vi "Measurement Logic.vi"(8 "error in":errorcluster, 9 "measurement configuration":T4={"config"="SI1", "BITFILE"=""}, 10 "measure call context in":refnum<class "Measure Call Context.lvclass">, 11 "user event out":refnum<user-event>) -> (0 "Error Out":errorcluster, 2 "measure call context out":refnum<class "Measure Call Context.lvclass">, 3 "measurement results":T1 {"BYTES ACQUIRED" format="%#.6p"})   [LabVIEW 2025, in "Automotive Vision.lvclass"]
doc: "Contains the core logic for executing the measurement."
uses:
  Automotive Vision.lvclass
  <vilib>/Plug-In SDKs/Measurements/Measure Call Context/Measure Call Context.lvclass
  <vilib>/rvi/interface/nirviCloseFPGA/nirviCloseFPGA.xnode
  Measurement Results.ctl
  <vilib>/FPGAPlugInAG/Dynamic/niLvFpga_Close_Dynamic.vi
  ttashjia/GSE/Host/Acq/GettingStarted_Acq_148X_Host.lvlib
  ttashjia/GSE/Host/Common/GettingStarted_Common_148X_Host.lvlib
  <instrlib>/FlexRIO/API/Host/v1/NI FlexRIO API v1.lvlib
  <vilib>/vision/Image Controls.llb/IMAQ Image.ctl
  <instrlib>/FlexRIO/CSI-2/v2/Common/Types/LLP Data Type.ctl
  <instrlib>/FlexRIO/CSI-2/v2/Common/NI CSI-2 API Common v2.lvlib
  <instrlib>/FlexRIO/API/Host/v1/NI FlexRIO/API/Wait for PoC Safe to Disconnect Channels Array.vi
  Measurement Configuration.ctl
panel:
  in  "Serial Channel (2nd Display)":fxp<+,3,3>
  in  "Serial Channel (1st Display)":fxp<+,3,3>
  in  "Acquired Serial Input Channel Data":T2(tab)
  out "Source Rate (fps)(1st Display)":dbl
  out "Update Rate (fps)(1st Display)":dbl
  out "1st channel display":T3(plugin-control)
  out "Bytes Acquired (1st Channel)":i64 format="%#.6p"
  out "Packets Logged (1st Channel)":i64
  out "Source Rate (fps)(2nd Display)":dbl
  out "Update Rate (fps)(2nd Display)":dbl
  out "2nd channel display":T3(plugin-control)
  out "Packets Logged (2nd Channel)":i64
  out "Bytes Acquired (2nd Channel)":i64 format="%#.6p"
  out "Acquisition In Progress":bool
  out "Acquisition Duration (s)":dbl format="%.1f"
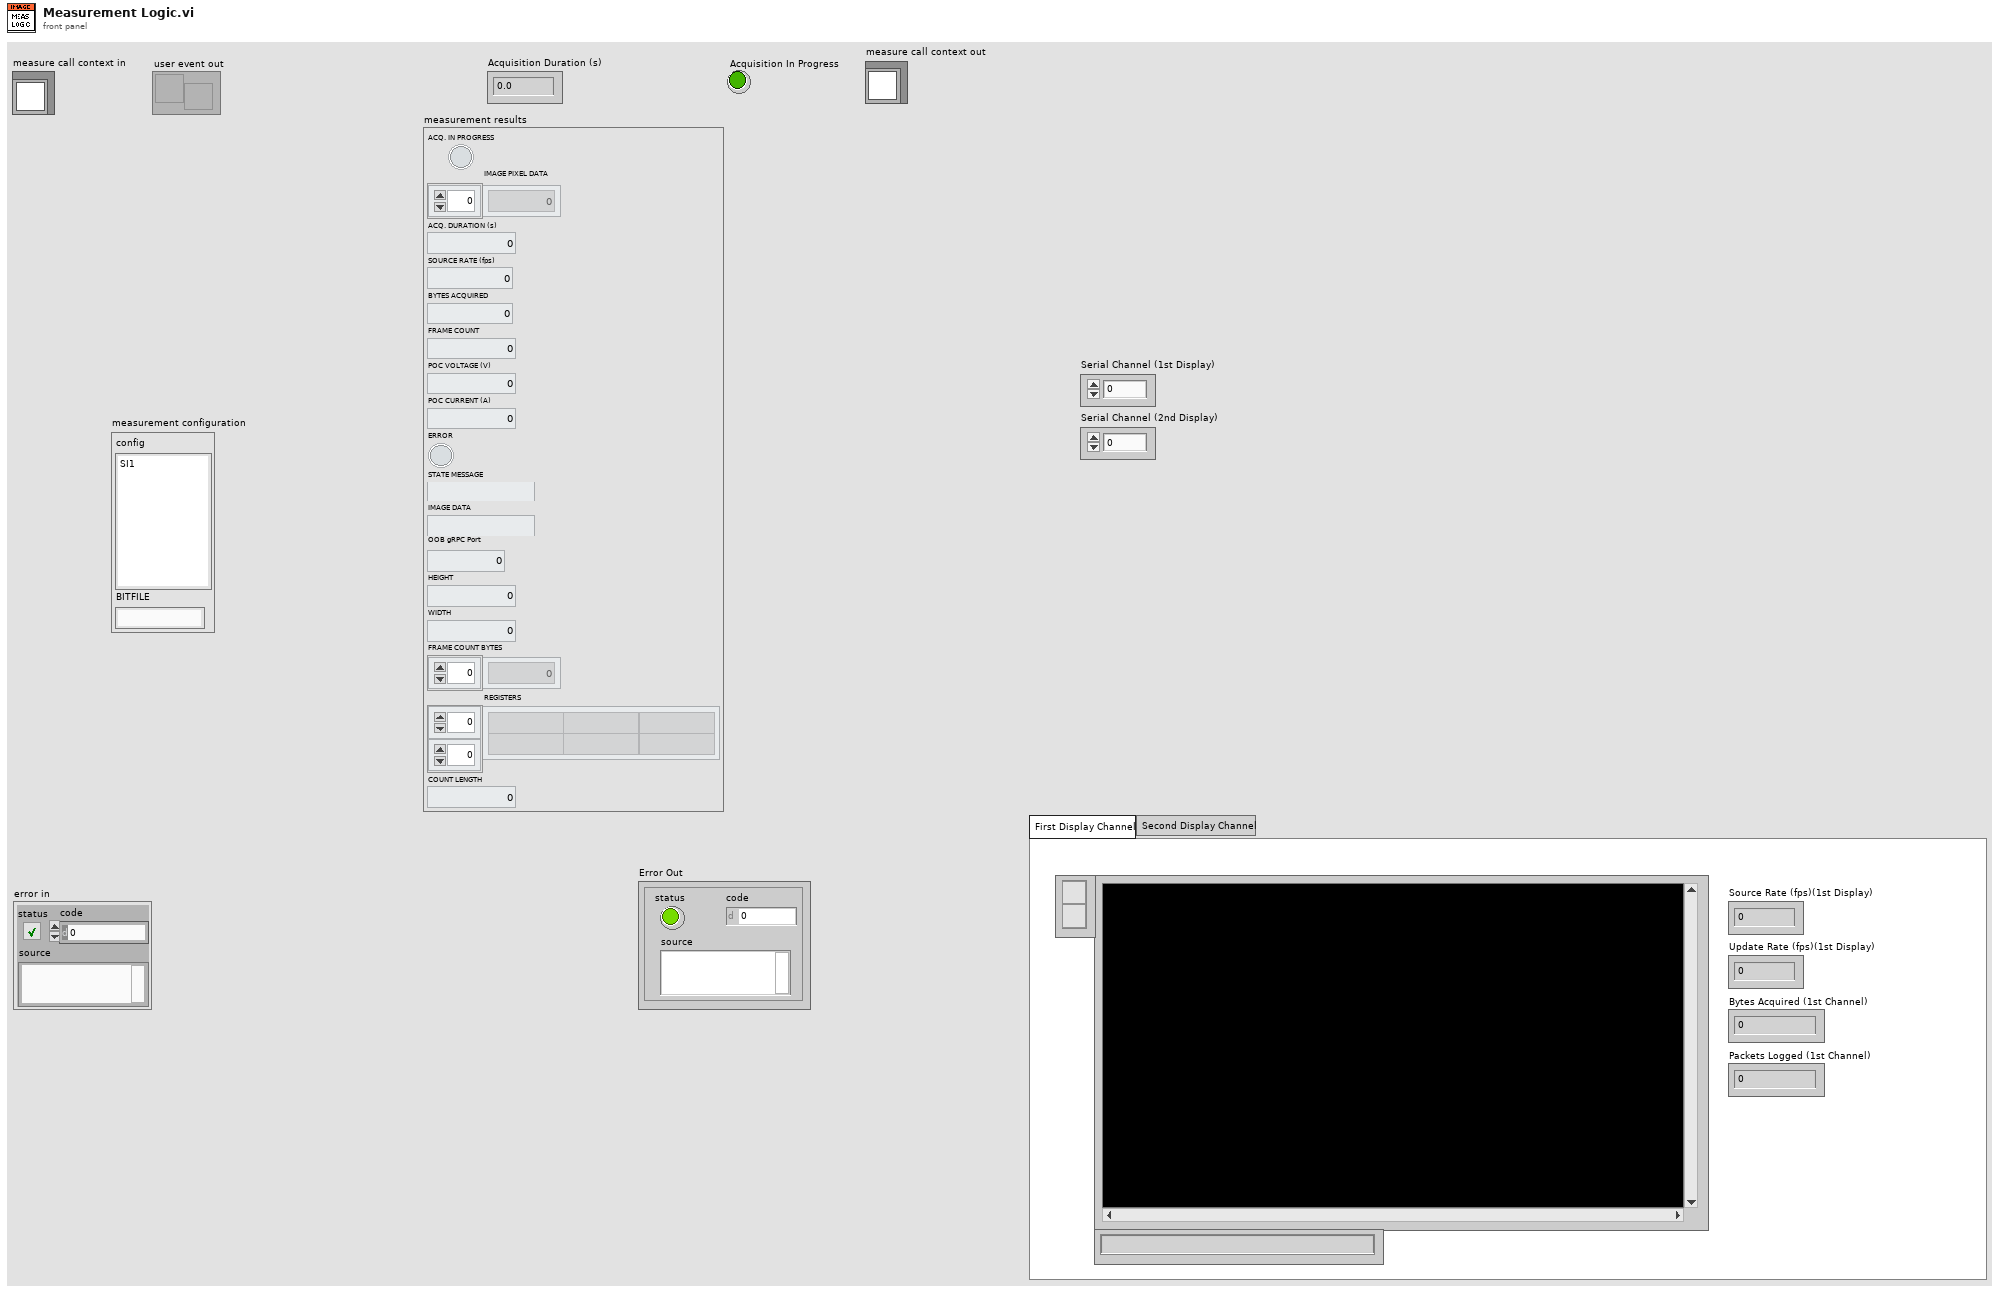
[diagram p1: front panel]
types:
  T1 = typedef "Automotive Vision.lvclass/Measurement Results.ctl" = cluster{"ACQ. IN PROGRESS":bool, "IMAGE PIXEL DATA":u32[], "ACQ. DURATION (s)":dbl, "SOURCE RATE (fps)":dbl, "BYTES ACQUIRED":u64, "FRAME COUNT":u64, "POC VOLTAGE (V)":dbl, "POC CURRENT (A)":dbl, "ERROR":bool, "STATE MESSAGE":string, "IMAGE DATA":string, "OOB gRPC Port":i32, "HEIGHT":u64, "WIDTH":u64, "FRAME COUNT BYTES":u32[], "REGISTERS":string[][], "COUNT LENGTH":u64}
  T2 = enum32{"First Display Channel", "Second Display Channel"}
  T3 = typedef "IMAQ Image.ctl" = refnum<image>
  T4 = typedef "Automotive Vision.lvclass/Measurement Configuration.ctl" = cluster{"config":string, "BITFILE":string}
  T5 = typedef "NI CSI-2 API Common v2.lvlib/LLP Data Type.ctl" = enum8{"Frame Start", "Frame End", "Line Start", "Line End", "End of Transmission", "Reserved 0", "Reserved 1", "Reserved 2", "Generic Short Packet 1", "Generic Short Packet 2", "Generic Short Packet 3", "Generic Short Packet 4", "Generic Short Packet 5", "Generic Short Packet 6", "Generic Short Packet 7", "Generic Short Packet 8", "Null", "Blanking Data", "Embedded 8-bit non Image Data", "Generic Long Packet 1", "Generic Long Packet 2", "Generic Long Packet 3", "Generic Long Packet 4", "Reserved 3", "YUV420 8-bit", "YUV420 10-bit", "Legacy YUV420 8-bit", "Reserved 4", "YUV420 8-bit Chroma Shifted", "YUV420 10-bit Chroma Shifted", "YUV422 8-bit", "YUV422 10-bit", "RGB444", "RGB555", "RGB565", "RGB666", "RGB888", "Reserved 5", "Reserved 6", "RAW 24", "RAW 6", "RAW 7", "RAW 8", "RAW 10", "RAW 12", "RAW 14", "RAW 16", "RAW 20", "User Defined 8-bit Data 1", "User Defined 8-bit Data 2", "User Defined 8-bit Data 3", "User Defined 8-bit Data 4", "User Defined 8-bit Data 5", "User Defined 8-bit Data 6", "User Defined 8-bit Data 7", "User Defined 8-bit Data 8", "USL Command", "Reserved 7", "Reserved 8", "Reserved 9", "Reserved 10", "Reserved 11", "Reserved 12", "LRTE EPD Spacer"}
  T6 = typedef "GettingStarted_Common_148X_Host.lvlib/Serial Channel Configuration.ctl" = cluster{"Serial Channel":string, "FPGA Display Parameters":T7, "RAW Display Parameters":cluster{"Interpretation":T8, "Bayer Parameters":cluster{"Pattern":i32, "Algorithm":i32, "Red Gain":dbl, "Green Gain":dbl, "Blue Gain":dbl}}}
  T7 = typedef "NI CSI-2 API FPGA v2.lvlib/Display Parameters.ctl" = cluster{"virtual channel":fxp<+,4,4>, "payload data type":T5, "frame skip count":u16, "line skip count":u8, "pixel skip count":fxp<+,5,5>}
  T8 = typedef "GettingStarted_Common_148X_Host.lvlib/RAW Interpretation for Display.ctl" = enum16{"Grayscale", "Bayer", "RGB", "YUV422", "YUV420", "Legacy YUV420"}
  T9 = typedef "Automotive Vision.lvclass/autovision_config.ctl" = cluster{"RIO Device":string, "Serial Channel":string, "SERDES Script":string, "POC Source":u32, "CSI-2 Data Source":u32, "Lane Count":u32, "Reference Clock":dbl, "Image Data Type":u32, "Interpretation":u32, "Pattern":u32, "Algorithm":u32, "Virtual Channel":u32, "Embedded Data":T10, "Registers":T12[], "Log Path":string}
  T10 = typedef "Automotive Vision.lvclass/embedded data.ctl" = cluster{"Pre-embedded Lines":dbl, "Pre-embedded Line Length":dbl, "Post-embedded Lines":dbl, "Post-embedded Line Length":dbl, "Frame Count":T11}
  T11 = typedef "Automotive Vision.lvclass/embedded data item.ctl" = cluster{"Line":dbl, "Offset":dbl, "Byte Count":dbl}
  T12 = typedef "Automotive Vision.lvclass/register.ctl" = cluster{"Name":string, "Device":u8, "Address":u16, "Min":u16, "Max":u16}
  T13 = typedef "GettingStarted_Common_148X_Host.lvlib/Serial Channel Display Parameters.ctl" = cluster{"images":cluster{"grayscale":T3, "color":T3}, "RAW parameters":cluster{"interpretation":T8, "bayer parameters":cluster{"pattern":i32, "algorithm":i32, "red gain":dbl, "green gain":dbl, "blue gain":dbl}}}
  T14 = cluster{"Acquisition In Progress":refnum<vi>, "Acquisition Duration (s)":refnum<vi>, "Bytes Acquired (1st Channel)":refnum<vi>}
  T15 = typedef "Event Messenger-bool.lvlib/))Channel.ctl" = refnum<queue>
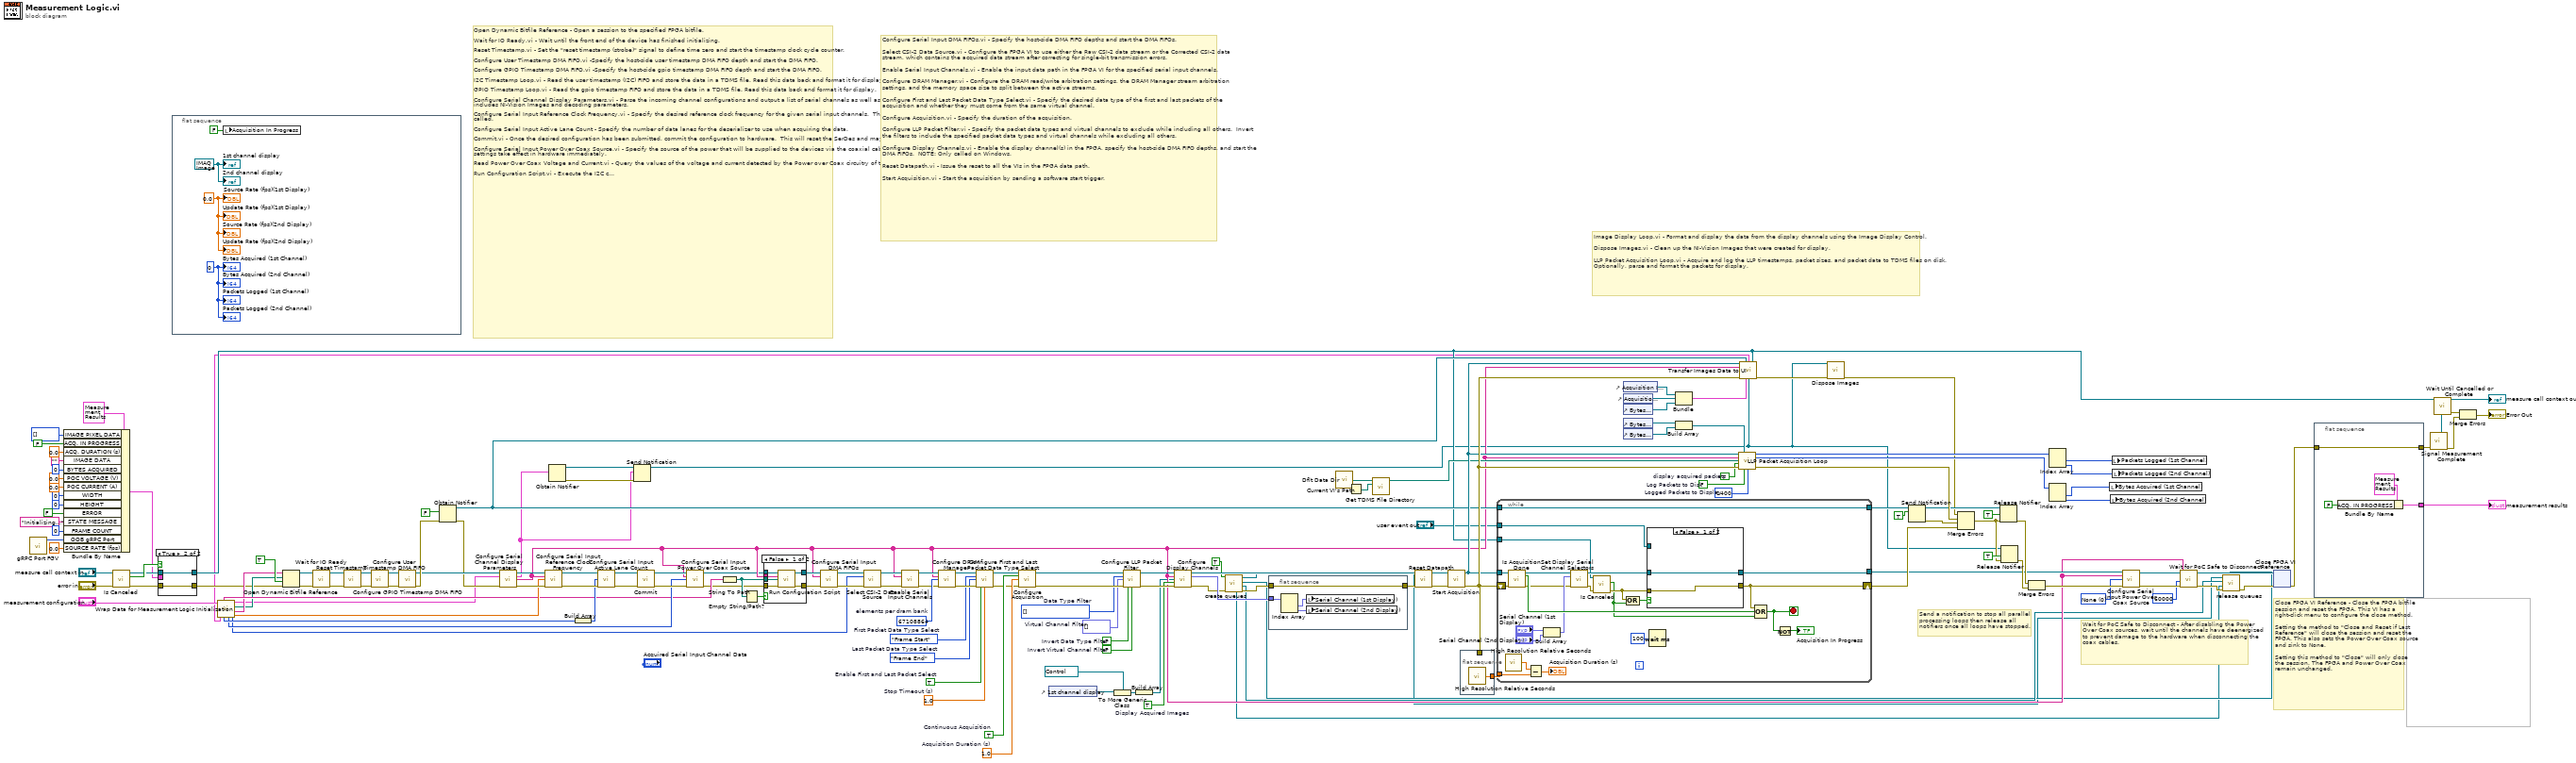
[diagram p0: block diagram]
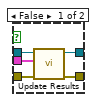
[diagram p2: hidden frame]
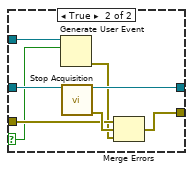
[diagram p3: hidden frame]
diagram:
  w84 = i64 1400  # Logged Packets to Display
  w112 = FALSE  # Log Packets to Disk
  w141 = FALSE  # Invert Virtual Channel Filter
  w142 = FALSE  # Invert Data Type Filter
  w143 = fxp<+,4,4>[] []  # Virtual Channel Filter
  w108 = TRUE  # Display Acquired Images
  w146 = T5[] [] items=["Frame Start", "Frame End", "Line Start", "Line End", "End of Transmission", "Reserved 0", "Reserved 1", "Reserved 2", "Generic Short Packet 1", "Generic Short Packet 2", "Generic Short Packet 3", "Generic Short Packet 4", "Generic Short Packet 5", "Generic Short Packet 6", "Generic Short Packet 7", "Generic Short Packet 8", "Null", "Blanking Data", "Embedded 8-bit non Image Data", "Generic Long Packet 1", "Generic Long Packet 2", "Generic Long Packet 3", "Generic Long Packet 4", "Reserved 3", "YUV420 8-bit", "YUV420 10-bit", "Legacy YUV420 8-bit", "Reserved 4", "YUV420 8-bit Chroma Shifted", "YUV420 10-bit Chroma Shifted", "YUV422 8-bit", "YUV422 10-bit", "RGB444", "RGB555", "RGB565", "RGB666", "RGB888", "Reserved 5", "Reserved 6", "RAW 24", "RAW 6", "RAW 7", "RAW 8", "RAW 10", "RAW 12", "RAW 14", "RAW 16", "RAW 20", "User Defined 8-bit Data 1", "User Defined 8-bit Data 2", "User Defined 8-bit Data 3", "User Defined 8-bit Data 4", "User Defined 8-bit Data 5", "User Defined 8-bit Data 6", "User Defined 8-bit Data 7", "User Defined 8-bit Data 8", "USL Command", "Reserved 7", "Reserved 8", "Reserved 9", "Reserved 10", "Reserved 11", "Reserved 12", "LRTE EPD Spacer"]  # Data Type Filter
  w149 = 1.0  # Acquisition Duration (s)
  w152 = TRUE  # Continuous Acquisition
  w131 = 1.0  # Stop Timeout (s)
  w132 = TRUE  # Enable First and Last Packet Select
  w129 = LLP_Data_Type."Frame End"  # Last Packet Data Type Select
  w130 = LLP_Data_Type."Frame Start"  # First Packet Data Type Select
  w66 = 0 items=["None", "Internal", "Auxiliary"] ("power over coax source")
  w85 = TRUE  # display acquired packets
  w158 = u32 67108864  # elements per dram bank
  # "Wait for PoC Safe to Disconnect - After disabling the Power Over Coax sources, wait until the channels have deenergized to prevent damage to the hardware when disconnecting the coax cables."
  # "Send a notification to stop all parallel processing loops then release all notifiers once all loops have stopped."
  # "Image Display Loop.vi - Format and display the data from the display channels using the Image Display Control.   \n\nDispose Images.vi - Clean up the NI-Vision Images that were created for display.\n\nLLP Packet Acquisition Loop.vi - Acquire and log the LLP timestamps, packet sizes, and packet data to TDMS files on disk.  Optionally, parse and format the packets for display."
  # "Configure Serial Input DMA FIFOs.vi - Specify the host-side DMA FIFO depths and start the DMA FIFOs.\n\nSelect CSI-2 Data Source.vi - Configure the FPGA VI to use either the Raw CSI-2 data stream or the Corrected CSI-2 data stream, which contains the acquired data stream after correcting for single-bit transmission errors.\n\nEnable Serial Input Channels.vi - Enable the input data path in the FPGA VI for the specified serial input channels.\n\nConfigure DRAM Manager.vi - Configure the DRAM read/write arbitration settings, the DRAM Manager stream arbitration settings, and the memory space size to split between the active streams.\n\nConfigure First and Last Packet Data Type Select.vi - Specify the desired data type of the first and last packets of the acquisition and whether they must come from the same virtual channel.\n\nConfigure Acquisition.vi - Specify the duration of the acquisition.\n\nConfigure LLP Packet Filter.vi - Specify the packet data types and virtual channels to exclude while including all others.  Invert the filters to include the specified packet data types and virtual channels while excluding all others.\n\nConfigure Display Channels.vi - Enable the display channel(s) in the FPGA, specify the host-side DMA FIFO depths, and start the DMA FIFOs.  NOTE: Only called on Windows. \n\nReset Datapath.vi - Issue the reset to all the VIs in the FPGA data path.\n\nStart Acquisition.vi - Start the acquisition by sending a software start trigger."
  # "Close FPGA VI Reference - Close the FPGA bitfile session and reset the FPGA. This VI has a right-click menu to configure the close method. \n\nSetting the method to \"Close and Reset if Last Reference\" will close the session and reset the FPGA. This also sets the Power Over Coax source and sink to None.\n\nSetting this method to \"Close\" will only close the session. The FPGA and Power Over Coax remain unchanged."
  # "Open Dynamic Bitfile Reference - Open a session to the specified FPGA bitfile.\n\nWait for IO Ready.vi - Wait until the front end of the device has finished initializing.\n\nReset Timestamp.vi - Set the \"reset timestamp (strobe)\" signal to define time zero and start the timestamp clock cycle counter.\n\nConfigure User Timestamp DMA FIFO.vi -Specify the host-side user timestamp DMA FIFO depth and start the DMA FIFO.\n\nConfigure GPIO Timestamp DMA FIFO.vi -Specify the host-side gpio timestamp DMA FIFO depth and start the DMA FIFO.\n\nI2C Timestamp Loop.vi - Read the user timestamp (I2C) FIFO and store the data in a TDMS file. Read this data back and format it for display.\n\nGPIO Timestamp Loop.vi - Read the gpio timestamp FIFO and store the data in a TDMS file. Read this data back and format it for display.\n\nConfigure Serial Channel Display Parameters.vi - Parse the incoming channel configurations and output a list of serial channels as well as a list of serial channel display parameters, which includes NI-Vision Images and decoding parameters.\n\nConfigure Serial Input Reference Clock Frequency.vi - Specify the desired reference clock frequency for the given serial input channels.  These settings do not take effect until Commit.vi is called.\n\nConfigure Serial Input Active Lane Count - Specify the number of data lanes for the deserializer to use when acquiring the data. \n\nCommit.vi - Once the desired configuration has been submitted, commit the configuration to hardware.  This will reset the SerDes and may cause GPIO lines to toggle. \n\nConfigure Serial Input Power Over Coax Source.vi - Specify the source of the power that will be supplied to the devices via the coaxial cables attached to the given serial input channels.  These settings take effect in hardware immediately.\n\nRead Power Over Coax Voltage and Current.vi - Query the values of the voltage and current detected by the Power over Coax circuitry of the given serial channels.\n\nRun Configuration Script.vi - Execute the I2C commands in the specified script file for the given serial channels.  The script is used to configure the serializer, deserializer, or other I2C slave device, such as the image sensor."
  n1 = call "gRPC Port FGV.vi"() -> ("Listening Port out"=w37:i32)  [unwired: 11 in]
  n2 = Bundle By Name(cluster=T1 {"ACQ. IN PROGRESS"=FALSE, "IMAGE PIXEL DATA"=[], "ACQ. DURATION (s)"=0.0, "SOURCE RATE (fps)"=0.0, "BYTES ACQUIRED"=0, "FRAME COUNT"=0, "POC VOLTAGE (V)"=0.0, "POC CURRENT (A)"=0.0, "ERROR"=FALSE, "STATE MESSAGE"="", "IMAGE DATA"="", "OOB gRPC Port"=0, "HEIGHT"=0, "WIDTH"=0, "FRAME COUNT BYTES"=[], "REGISTERS"=[], "COUNT LENGTH"=0} ("Measurement Results"), "IMAGE PIXEL DATA"=u32[] [], "ACQ. IN PROGRESS"=FALSE, "ACQ. DURATION (s)"=0.0, "IMAGE DATA"="", "BYTES ACQUIRED"=u64 0, "POC VOLTAGE (V)"=0.0, "POC CURRENT (A)"=0.0, "WIDTH"=u64 0, "HEIGHT"=u64 0, "ERROR"=FALSE, "STATE MESSAGE"="Initializing...", "FRAME COUNT"=u64 0, "OOB gRPC Port"=w37, "SOURCE RATE (fps)"=0.0) -> (w33:T1)
  n3 = call <vilib>:"Is Canceled.vi"("error in"="error in", "measure call context in"="measure call context in") -> ("error out"=w36:errorcluster, "is canceled?"=w35:bool, "measure call context out"=w34:refnum<class "Measure Call Context.lvclass">)  [unwired: 7 in]
  n4 = case shown="True" w35 {
    tunnel: w33 -> [w167 _]
    tunnel: [w166 w169] -> w30
    tunnel: w34 -> [w165 w168]
    tunnel: w36 -> [w164 w169]
    tunnel: [w163 w168] -> w15
    frame False {
      n5 = call <vilib>:"Update Results.vi"("error in"=w164, "measurement results"=w167, "measure call context in"=w165) -> ("error out"=w166:errorcluster, "measure call context out"=w163:refnum<class "Measure Call Context.lvclass">)  [unwired: 7 in]
    }
    frame True {
    }
  }
  n6 = flat-sequence {
    frame #0 {
      w171 = i64 0 ("Number of Packets Acquired (1st Channel)")
      w172 = 0.0 ("display fps (2nd display)")
      w173 = T3 refnum ("first channel display")
      n7 = local write "Acquisition In Progress"(FALSE ("Acquisition In Progress")) -> ()
      "1st channel display" <- w173
      "2nd channel display" <- w173
      "Update Rate (fps)(1st Display)" <- w172
      "Update Rate (fps)(2nd Display)" <- w172
      "Packets Logged (1st Channel)" <- w171
      "Packets Logged (2nd Channel)" <- w171
      "Source Rate (fps)(1st Display)" <- w172
      "Source Rate (fps)(2nd Display)" <- w172
      "Bytes Acquired (1st Channel)" <- w171
      "Bytes Acquired (2nd Channel)" <- w171
    }
  }
  n8 = call "Wrap Data for Measurement Logic Initialization.vi"("measurement configuration"="measurement configuration") -> ("REF. CLOCK  (Hz)"=w56:dbl, "RIO HANDLER"=w52:string, "CSI-2 DATA SOURCE"=w57:u32, "Serial Input Configuration"=w45:T6[], "POC SOURCE"=w58:u32, "appended path"=w51:path, "SI ACTIVE LANE CNT"=w59:u32, "PATH TO CONFIGURATION SCRIPT"=w55:string, "config"=w9:T9)  [unwired: 2 in]
  n9 = Open Dynamic Bitfile Reference(0:w52, 1:w51, 2:TRUE ("Run When Loaded"), 3:w30) -> (5:w144:refnum<k20>, 8:w46:errorcluster)  [unwired: 1 in]
  n10 = call <instrlib>:"Wait for IO Ready.vi"("fpga interface in"=w144, "error in"=w46) -> ("fpga interface out"=w105:refnum<k20>, "error out"=w106:errorcluster)  [unwired: 10 in, 2 out]
  n11 = call "Reset Timestamp.vi"("fpga interface in"=w105, "error in (no error)"=w106) -> ("fpga interface out"=w95:refnum<k20>, "error out"=w94:errorcluster)  [unwired: 12 in]
  n12 = call "Configure User Timestamp DMA FIFO.vi"("fpga interface in"=w95, "error in (no error)"=w94) -> ("fpga interface out"=w93:refnum<k20>, "error out"=w92:errorcluster)  [unwired: 12 in]
  n13 = call "Configure GPIO Timestamp DMA FIFO.vi"("fpga interface in"=w93, "error in (no error)"=w92) -> ("fpga interface out"=w89:refnum<k20>, "error out"=w91:errorcluster)  [unwired: 12 in]
  n14 = Obtain Notifier(notification data type=FALSE ("result"), error in (no error)=w91) -> (notifier out=w77:refnum<notifier>, error out=w88:errorcluster)  [unwired: 2 in, 1 out]
  n15 = call "Configure Serial Channel Display Parameters.vi"("fpga interface in"=w89, "serial channel configurations"=w45, "error in (no error)"=w88) -> ("fpga interface out"=w121:refnum<k20>, "serial channel display parameters"=w74:T13[], "serial channels"=w44:string[], "error out"=w120:errorcluster)  [unwired: 9 in]
  n16 = call "Configure Serial Input Reference Clock Frequency.vi"("fpga interface in"=w121, "serial input channels"=w44, "serial input reference clock frequency (Hz)"=w56, "error in (no error)"=w120) -> ("fpga interface out"=w82:refnum<k20>, "error out"=w81:errorcluster)  [unwired: 10 in]
  n17 = Obtain Notifier(notification data type=w74) -> (notifier out=w76:refnum<notifier>, error out=w75:errorcluster)  [unwired: 3 in, 1 out]
  n18 = Build Array(w59) -> (w78:u32[])
  n19 = call "Configure Serial Input Active Lane Count.vi"("fpga interface in"=w82, "serial input active lane counts"=w78, "error in (no error)"=w81) -> ("fpga interface out"=w80:refnum<k20>, "error out"=w79:errorcluster)  [unwired: 11 in]
  n20 = Send Notification(notification=w74, notifier=w76, error in (no error)=w75) -> (notifier out=w14:refnum<notifier>)  [unwired: 1 out]
  n21 = call <instrlib>:"Commit.vi"("fpga interface in"=w80, "error in"=w79) -> ("fpga interface out"=w147:refnum<k20>, "error out"=w148:errorcluster)  [unwired: 12 in]
  n22 = call "Configure Serial Input Power Over Coax Source.vi"("fpga interface in"=w147, "serial input channels"=w44, "power over coax source"=w58, "error in (no error)"=w148) -> ("fpga interface out"=w39:refnum<k20>, "error out"=w38:errorcluster)  [unwired: 9 in, 1 out]
  n23 = String To Path(string=w55) -> (path=w54:path)
  n24 = Empty String/Path?(string/path=w54) -> (empty?=w107:bool)
  n25 = case shown="False" w107 {
    tunnel: [w179 w180] -> w156
    tunnel: [w178 w181] -> w151
    tunnel: w38 -> [w177 w180]
    tunnel: w39 -> [w176 w181]
    tunnel: w44 -> [w175 _]
    tunnel: w54 -> [w174 _]
    frame False {
      n26 = call "Run Configuration Script.vi"("fpga interface in"=w176, "serial channels"=w175, "configuration script"=w174, "error in (no error)"=w177) -> ("fpga interface out"=w178:refnum<k20>, "error out"=w179:errorcluster)  [unwired: 10 in]
    }
    frame True {
    }
  }
  n27 = call "Configure Serial Input DMA FIFOs.vi"("fpga interface in"=w151, "serial channels"=w44, "error in (no error)"=w156) -> ("fpga interface out"=w140:refnum<k20>, "error out"=w137:errorcluster)  [unwired: 11 in]
  n28 = call "Select CSI-2 Data Source.vi"("fpga interface in"=w140, "csi-2 data source"=w57, "error in (no error)"=w137) -> ("fpga interface out"=w139:refnum<k20>, "error out"=w138:errorcluster)  [unwired: 11 in]
  n29 = call "Enable Serial Input Channels.vi"("fpga interface in"=w139, "serial input channels"=w44, "error in (no error)"=w138) -> ("fpga interface out"=w150:refnum<k20>, "error out"=w157:errorcluster)  [unwired: 11 in]
  n30 = call "Configure DRAM Manager.vi"("fpga interface in"=w150, "serial channels"=w44, "elements per dram bank"=w158, "error in (no error)"=w157) -> ("fpga interface out"=w133:refnum<k20>, "error out"=w136:errorcluster)  [unwired: 10 in]
  n31 = call "Configure First and Last Packet Data Type Select.vi"("fpga interface in"=w133, "first packet data type select"=w130, "last packet data type select"=w129, "error in (no error)"=w136, "enable first and last packet select"=w132, "stop timeout (s)"=w131) -> ("fpga interface out"=w134:refnum<k20>, "error out"=w135:errorcluster)  [unwired: 8 in]
  n32 = call "Configure Acquisition.vi"("fpga interface in"=w134, "continuous acquisition (T)"=w152, "acquisition duration (s)"=w149, "error in (no error)"=w135) -> ("fpga interface out"=w153:refnum<k20>, "error out"=w154:errorcluster)  [unwired: 10 in]
  n33 = control-ref of="1st channel display"() -> (w41:refnum<vi>)
  n34 = To More Generic Class(target class=refnum<vi> refnum ("image display reference"), reference=w41) -> (generic class reference=w43:refnum<vi>)
  n35 = call "Configure LLP Packet Filter.vi"("fpga interface in"=w153, "data type filter"=w146, "virtual channel filter"=w143, "error in (no error)"=w154, "invert data type filter"=w142, "invert virtual channel filter"=w141) -> ("fpga interface out"=w122:refnum<k20>, "error out"=w119:errorcluster)  [unwired: 8 in]
  n36 = Build Array(w43) -> (w40:refnum<vi>[])
  n37 = call "Configure Display Channels.vi"("fpga interface in"=w122, "serial channels"=w44, "display references in"=w40, "enable image display"=w108, "error in (no error)"=w119) -> ("fpga interface out"=w118:refnum<k20>, "display serial channels"=w117:fxp<+,3,3>[], "error out"=w10:errorcluster)  [unwired: 7 in, 1 out]
  n38 = call "create queues.vi"("error in (no error)"=w10, "create if not found? (T)"=TRUE) -> ("error out"=w8:errorcluster, "i2c queue out"=w4:refnum<queue>, "power monitor queue out"=w3:refnum<queue>, "image queue out"=w2:refnum<queue>, "register monitor queue out"=w1:refnum<queue>)  [unwired: 5 in]
  n39 = flat-sequence {
    tunnel: w117 -> [w183]
    tunnel: w8 -> [w182]
    tunnel: [w182] -> w116
    frame #0 {
      n40 = Index Array(array=w183) -> (element #1=w185:fxp<+,3,3>, element #2=w184:fxp<+,3,3>)  [unwired: 2 in]
      n41 = local write "Serial Channel (1st Display)"(w185) -> ()
      n42 = local write "Serial Channel (2nd Display)"(w184) -> ()
    }
  }
  n43 = call <vilib>:"Dflt Data Dir.vi"() -> ("App:Default Data Directory"=w53:path)
  n44 = Current VI's Path() -> (path=w125:path)
  n45 = call "Get TDMS File Directory.vi"("tdms file directory in"=w53, "calling vi path"=w125) -> ("tdms file directory out"=w87:path)  [unwired: 13 in]
  n46 = call "Reset Datapath.vi"("fpga interface in"=w118, "error in (no error)"=w116) -> ("fpga interface out"=w155:refnum<k20>, "error out"=w90:errorcluster)  [unwired: 12 in]
  n47 = call "Start Acquisition.vi"("fpga interface in"=w155, "error in (no error)"=w90) -> ("fpga interface out"=w103:refnum<k20>, "error out"=w104:errorcluster)  [unwired: 12 in]
  n48 = flat-sequence {
    tunnel: [w186] -> w126
    tunnel: w104 -> [_]
    frame #0 {
      n49 = call <vilib>:"High Resolution Relative Seconds.vi"() -> ("relative seconds"=w186:dbl)
    }
  }
  n50 = while {
    shift-right: [w190] -> w83
    shift-left: w104 -> [w201]
    tunnel: w103 -> [w203]
    tunnel: w126 -> [w207]
    tunnel: w77 -> [w200]
    tunnel: [w200] -> w100
    tunnel: [w191] -> w69
    tunnel: w15 -> [w197]
    tunnel: "user event out" -> [w187]
    stop <- w202 stop-if-true
    n51 = call <vilib>:"High Resolution Relative Seconds.vi"() -> ("relative seconds"=w208:dbl)
    n52 = call "Is Acquisition Done.vi"("fpga interface in"=w203, "error in (no error)"=w201) -> ("fpga interface out"=w193:refnum<k20>, "acquisition done"=w210:bool, "error out"=w192:errorcluster)  [unwired: 11 in]
    n53 = Subtract(x=w208, y=w207) -> (x-y=→"Acquisition Duration (s)":dbl)
    n54 = Build Array("Serial Channel (1st Display)", "Serial Channel (2nd Display)") -> (w204:fxp<+,3,3>[])
    n55 = call "Set Display Serial Channel Selectors.vi"("fpga interface in"=w193, "display serial channel selectors"=w204, "error in (no error)"=w192) -> ("fpga interface out"=w198:refnum<k20>, "error out"=w199:errorcluster)  [unwired: 11 in]
    n56 = call <vilib>:"Is Canceled.vi"("error in"=w199, "measure call context in"=w197) -> ("error out"=w195:errorcluster, "is canceled?"=w189:bool)  [unwired: 7 in, 1 out]
    n57 = Compound Arithmetic op=OR(w195, w189) -> (w188:bool)
    n58 = case shown="False" w188 {
      selector: w188 -> [_ w214]
      tunnel: [w212 w217] -> w190
      tunnel: w195 -> [w212 w216]
      tunnel: [w211 w219] -> w191
      tunnel: w198 -> [w211 w218]
      tunnel: w187 -> [_ w215]
      frame False {
      }
      frame True {
        n59 = Generate User Event(user event=w215, event data cluster=w214) -> (error out=w213:errorcluster)  [unwired: 2 in, 1 out]
        n60 = call "Stop Acquisition.vi"("fpga interface in"=w218) -> ("fpga interface out"=w219:refnum<k20>, "error out"=w220:errorcluster)  [unwired: 13 in]
        n61 = Merge Errors(w216, w220, w213) -> (w217:errorcluster)
      }
    }
    n62 = Wait (ms)(milliseconds to wait=u32 100) -> ()  [unwired: 1 out]
    n63 = Compound Arithmetic op=OR(w190, w210, w189) -> (w202:bool)
    n64 = Not(x=w202) -> (.not. x?=→"Acquisition In Progress":bool)
  }
  n65 = control-ref of="Acquisition In Progress"() -> (w50:refnum<vi>)
  n66 = control-ref of="Acquisition Duration (s)"() -> (w49:refnum<vi>)
  n67 = control-ref of="Bytes Acquired (1st Channel)"() -> (w48:refnum<vi>)
  n68 = control-ref of="Bytes Acquired (1st Channel)"() -> (w128:refnum<vi>)
  n69 = control-ref of="Bytes Acquired (2nd Channel)"() -> (w127:refnum<vi>)
  n70 = Bundle("Acquisition In Progress"=w50, "Acquisition Duration (s)"=w49, "Bytes Acquired (1st Channel)"=w48) -> (w47:T14)  [unwired: 1 in]
  n71 = Build Array(w128, w127) -> (w124:refnum<vi>[])
  n72 = call "LLP Packet Acquisition Loop.vi"("fpga interface in"=w103, "bytes acquired references"=w124, "Serial Channels"=w44, "tdms file directory"=w87, "display acquired packets"=w85, "error in"=w104, "log to disk"=w112, "num packets to read"=w84) -> ("number of packets acquired"=w123:i64[], "number of bytes acquired"=w111:i64[], "error out"=w101:errorcluster)  [unwired: 4 in, 1 out]
  n73 = call "Transfer Images Data to UI.vi"("fpga interface in"=w103, "'stop' notifier"=w77, "Auto Vision Config"=w9, "measure call context in"=w15, "Active Channel"=w44, "error in"=w104, "References"=w47, "raw display notifier"=w14) -> ("error out"=w113:errorcluster)  [unwired: 6 in, 1 out]
  n74 = call "Dispose Images.vi"("raw display notifier"=w14, "error in (no error)"=w113) -> ("error out"=w86:errorcluster)  [unwired: 13 in]
  n75 = Send Notification(notification=TRUE, notifier=w100) -> (notifier out=w99:refnum<notifier>, error out=w98:errorcluster)  [unwired: 1 in]
  n76 = Merge Errors(w86, w101, w98, w83) -> (w72:errorcluster)
  n77 = Release Notifier(notifier=w99, force destroy? (F)=TRUE, error in (no error)=w72) -> (error out=w71:errorcluster)  [unwired: 2 out]
  n78 = Release Notifier(notifier=w14, force destroy? (F)=TRUE, error in (no error)=w72) -> (error out=w70:errorcluster)  [unwired: 2 out]
  n79 = Merge Errors(w71, w70) -> (w68:errorcluster)
  n80 = Index Array(array=w123) -> (element #1=w115:i64, element #2=w114:i64)  [unwired: 2 in]
  n81 = Index Array(array=w111) -> (element #1=w110:i64, element #2=w109:i64)  [unwired: 2 in]
  n82 = local write "Bytes Acquired (1st Channel)"(w110) -> ()
  n83 = local write "Bytes Acquired (2nd Channel)"(w109) -> ()
  n84 = local write "Packets Logged (1st Channel)"(w115) -> ()
  n85 = local write "Packets Logged (2nd Channel)"(w114) -> ()
  n86 = call "Configure Serial Input Power Over Coax Source.vi"("fpga interface in"=w69, "serial input channels"=w44, "power over coax source"=w66, "error in (no error)"=w68) -> ("fpga interface out"=w64:refnum<k20>, "error out"=w65:errorcluster)  [unwired: 9 in, 1 out]
  n87 = call-poly <instrlib>:"Wait for PoC Safe to Disconnect.vi"("error in"=w65, "Timeout (ms)"=60000 ("Wait for Safe to Disconnect Timeout (ms)"), "Channels"=w44, "fpga interface in"=w64) -> ("error out"=w6:errorcluster, "fpga interface out"=w67:refnum<k20>)  [unwired: 6 in]
  n88 = call "release queues.vi"("power monitor queue out"=w3, "error in (no error)"=w6, "register monitor queue out"=w1, "i2c queue out"=w4, "image queue out"=w2) -> ("error out"=w5:errorcluster)  [unwired: 6 in]
  n89 = xnode ("Close FPGA VI Reference")("FPGA VI Reference In"=w67, "error in"=w5) -> ("error out"=w60:errorcluster)
  n90 = flat-sequence {
    tunnel: [w223] -> w61
    tunnel: w60 -> [w221]
    tunnel: [w221] -> w13
    frame #0 {
      n91 = Bundle By Name(cluster=T1 {"ACQ. IN PROGRESS"=FALSE, "IMAGE PIXEL DATA"=[], "ACQ. DURATION (s)"=0.0, "SOURCE RATE (fps)"=0.0, "BYTES ACQUIRED"=0, "FRAME COUNT"=0, "POC VOLTAGE (V)"=0.0, "POC CURRENT (A)"=0.0, "ERROR"=FALSE, "STATE MESSAGE"="", "IMAGE DATA"="", "OOB gRPC Port"=0, "HEIGHT"=0, "WIDTH"=0, "FRAME COUNT BYTES"=[], "REGISTERS"=[], "COUNT LENGTH"=0} ("Measurement Results"), "ACQ. IN PROGRESS"=FALSE) -> (w223:T1)
    }
  }
  n92 = call "Signal Measurement Complete.vi"("error in (no error)"=w13) -> ("error out"=w160:errorcluster, "done channel"=w161:T15)  [unwired: 9 in]
  n93 = call "Wait Until Cancelled or Complete.vi"("done channel"=w161, "measure call context in"=w15) -> ("error out"=w159:errorcluster, "measure call context out"=→"measure call context out":refnum<class "Measure Call Context.lvclass">)  [unwired: 8 in]
  n94 = Merge Errors(w159, w160) -> (→"Error Out":errorcluster)
  "measurement results" <- w61
